vi "Display Module Get Image ROI.vi"(7 "Image Ref":T1, 11 "Error In":errorcluster) -> (4 "H Offset":i32, 6 "V Offset":i32, 8 "H Width":i32, 10 "V Width":i32, 15 "Error Out":errorcluster)   [LabVIEW 2020]
uses:
  <vilib>/vision/Image Controls.llb/IMAQ Image.ctl
  Display Module Custom Controls/ROI Descriptor.ctl
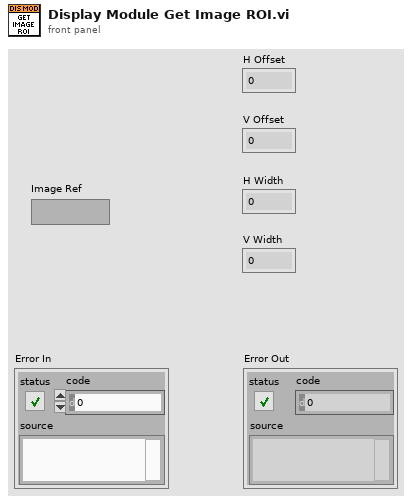
[diagram p1: front panel]
types:
  T1 = typedef "IMAQ Image.ctl" = refnum<image>
  T2 = typedef "ROI Descriptor.ctl" = cluster{"Global Rectangle":i32[], "Contours":cluster{"Contour Type":u32, "ROI Type":u32, "Points":i32[]}[]}
  T3 = typedef "Camera IMAQ Key Info.ctl" = cluster{"Frame":u32, "Sensor Height":i32, "Sensor Width":i32, "ROI Height":i32, "ROI Width":i32, "ROI Enable?":bool, "Bit per Pixel":u8}
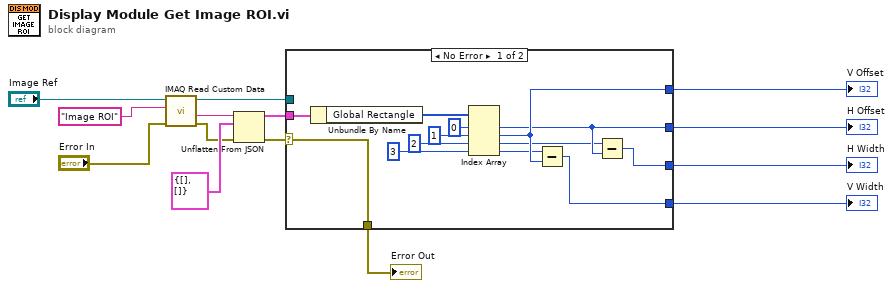
[diagram p0: block diagram]
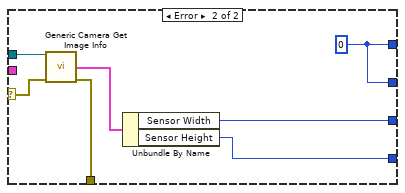
[diagram p2: hidden frame]
diagram:
  n1 = call "IMAQ Read Custom Data"("error in (no error)"="Error In", "Key"="Image ROI", "Image"="Image Ref") -> ("error out"=w4:errorcluster, "Custom Data Out"=w5:string, "Image (duplicate)"=w8:T1)  [unwired: 6 in]
  n2 = Unflatten From JSON(JSON string=w5, type and defaults=T2 {"Global Rectangle"=[], "Contours"=[]} ("Image ROI Descriptor"), error in (no error)=w4) -> (value=w2:T2, error out=w3:errorcluster)  [unwired: 4 in]
  n3 = case shown="No Error" w3 {
    selector: w3 -> [w15 w28]
    tunnel: [w27 w30] -> w14
    tunnel: [w26 w30] -> w13
    tunnel: [w25 w32] -> w12
    tunnel: [w24 w31] -> w11
    tunnel: w8 -> [_ w34]
    tunnel: [w15 w29] -> w1
    tunnel: w2 -> [w16 _]
    frame No Error {
      n4 = Unbundle By Name(w16) -> ("Global Rectangle"=w23:i32[])
      n5 = Index Array(array=w23, index #1=0 ("index"), index #2=1 ("index"), index #3=2 ("index"), index #4=3 ("index")) -> (element #1=w26:i32, element #2=w27:i32, element #3=w17:i32, element #4=w18:i32)
      n6 = Subtract(x=w18, y=w27) -> (x-y=w25:i32)
      n7 = Subtract(x=w17, y=w26) -> (x-y=w24:i32)
    }
    frame Error {
      w30 = 0
      n8 = call "Generic Camera Get Image Info.vi"("Image Ref"=w34, "Error In"=w28) -> ("Camera Image Info"=w33:T3, "Error Out"=w29:errorcluster)  [unwired: 11 in, 1 out]
      n9 = Unbundle By Name(w33) -> ("Sensor Width"=w31:i32, "Sensor Height"=w32:i32)
    }
  }
  "V Offset" <- w14
  "V Width" <- w12
  "H Width" <- w11
  "H Offset" <- w13
  "Error Out" <- w1
